vi "ex_readLines.vi"(0 "line string":string, 1 "# Lines to Skip":i32=2) -> (3 "Channel Names":string, 4 "Data":string)   [LabVIEW 2017]
panel:
  out "offset past match 2":i32
  out "offset past match":i32
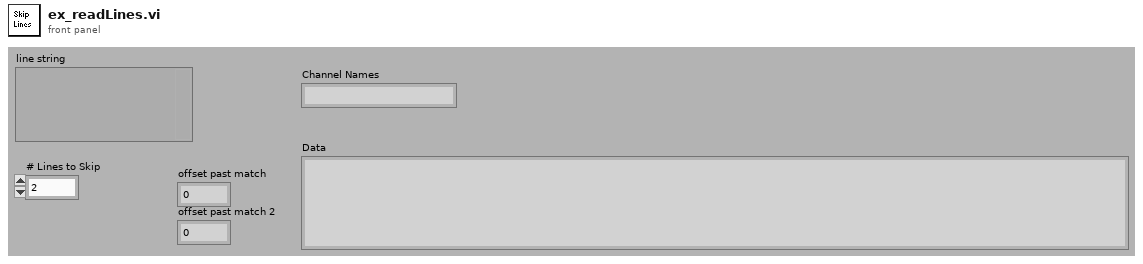
[diagram p1: front panel]
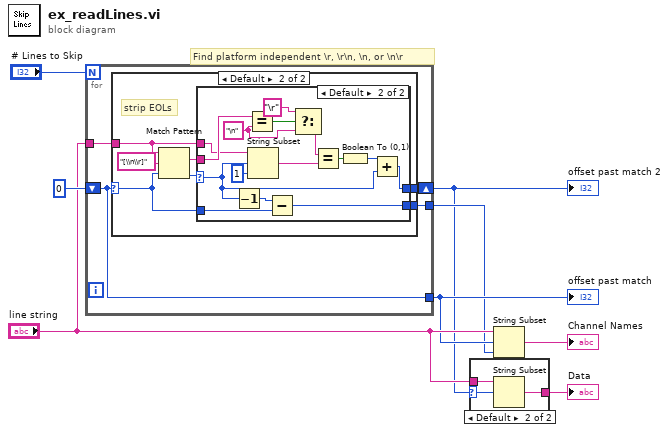
[diagram p0: block diagram]
diagram:
  # "Find platform independent \\r, \\r\\n, \\n, or \\n\\r"
  n1 = for {
    N: "# Lines to Skip" -> [_]
    tunnel: "line string" -> [w12]
    shift-right: [w11] -> w2
    shift-left: 0 ("offset past match") -> [w10]
    tunnel: [w10] -> w4
    tunnel: [w9] -> w3
    n2 = case shown="Default" w10 {
      selector: w10 -> [w13 w15]
      tunnel: w12 -> [_ w18]
      tunnel: [w13 w17] -> w11
      tunnel: [_ w14] -> w9
      frame -1 {
      }
      frame Default {
        # "strip EOLs"
        n3 = Match Pattern(string=w18, regular expression="[\\n\\r]", offset (0)=w15) -> (match substring=w19:string, offset past match=w16:i32)  [unwired: 2 out]
        n4 = case shown="Default" w16 {
          selector: w16 -> [w21 w25]
          tunnel: w19 -> [_ w36]
          tunnel: w18 -> [_ w31]
          tunnel: [w21 w27] -> w17
          tunnel: w15 -> [_ w23]
          tunnel: [_ w22] -> w14
          frame -1 {
          }
          frame Default {
            w33 = "\n"
            n5 = Decrement(x=w25) -> (x-1=w24:i32)
            n6 = Equal?(x=w36, y=w33) -> (x = y?=w35:bool)
            n7 = String Subset(string=w31, offset (0)=w25, length (rest)=1 ("length (rest)")) -> (substring=w29:string)
            n8 = Subtract(x=w24, y=w23) -> (x-y=w22:i32)
            n9 = Select(t="\r", s=w35, f=w33) -> (s? t:f=w30:string)
            n10 = Equal?(x=w30, y=w29) -> (x = y?=w28:bool)
            n11 = Boolean To (0,1)(Boolean=w28) -> (0, 1=w26:i16)
            n12 = Add(x=w26, y=w25) -> (x+y=w27:i32)
          }
        }
      }
    }
  }
  "offset past match" <- w4
  "offset past match 2" <- w2
  n13 = case shown="Default" w2 {
    selector: w2 -> [_ w38]
    tunnel: "line string" -> [_ w39]
    tunnel: [_ w37] -> w1
    frame -1 {
    }
    frame Default {
      n14 = String Subset(string=w39, offset (0)=w38) -> (substring=w37:string)  [unwired: 1 out]
    }
  }
  "Data" <- w1
  n15 = String Subset(string="line string", offset (0)=w4, length (rest)=w3) -> (substring=→"Channel Names":string)
